vi "SRXConfigVoltageCompensation.vi"(3 "error in":errorcluster, 4 "RobotMotors":T16={"DriveRightPrimary"={"DeviceStatus"={"status"=FALSE, "code"=0, "source"=""}, "Type"=enum."PWM", "PWM"={"PWM Channel"=enum."PWM 1", "DeadBand"={"Name"="", "maxPositivePwm"=0, "minPositivePwm"=0, "centerPwm"=0, "maxNegativePwm"=0, "minNegativePwm"=0, "angularRange"=0}}, "CAN"={"Device Number"=0, "SetOutput VI Ref"=variant(enum8{"Percent VBus", "Current", "Speed", "Position", "Voltage"} enum."Percent VBus"), "GetOutput VI Ref"=variant(refnum<k1> refnum), "Enable VI Ref"=variant(dbl 12.0), "Disable VI Ref"=variant(enum8{"Percent VBus", "Speed", "Position", "Slave", "Unchanged / Invalid", "Voltage Compensation", "Current", "Motion Profile"} enum."Percent VBus"), "Data"=variant}, "Invert"=FALSE, "DIO PWM"={"PWM \"Enable\" Channel"=enum."Invalid", "DIOChannel"=enum."Invalid", "PWM Rate"=0.0}}, "DriveRightSecondary"={"DeviceStatus"={"status"=FALSE, "code"=0, "source"=""}, "Type"=enum."PWM", "PWM"={"PWM Channel"=enum."PWM 1", "DeadBand"={"Name"="", "maxPositivePwm"=0, "minPositivePwm"=0, "centerPwm"=0, "maxNegativePwm"=0, "minNegativePwm"=0, "angularRange"=0}}, "CAN"={"Device Number"=0, "SetOutput VI Ref"=variant(enum8{"Percent VBus", "Current", "Speed", "Position", "Voltage"} enum."Percent VBus"), "GetOutput VI Ref"=variant(refnum<k1> refnum), "Enable VI Ref"=variant(dbl 12.0), "Disable VI Ref"=variant(enum8{"Percent VBus", "Speed", "Position", "Slave", "Unchanged / Invalid", "Voltage Compensation", "Current", "Motion Profile"} enum."Percent VBus"), "Data"=variant}, "Invert"=FALSE, "DIO PWM"={"PWM \"Enable\" Channel"=enum."Invalid", "DIOChannel"=enum."Invalid", "PWM Rate"=0.0}}, "DriveLeftPrimary"={"DeviceStatus"={"status"=FALSE, "code"=0, "source"=""}, "Type"=enum."PWM", "PWM"={"PWM Channel"=enum."PWM 1", "DeadBand"={"Name"="", "maxPositivePwm"=0, "minPositivePwm"=0, "centerPwm"=0, "maxNegativePwm"=0, "minNegativePwm"=0, "angularRange"=0}}, "CAN"={"Device Number"=0, "SetOutput VI Ref"=variant(enum8{"Percent VBus", "Current", "Speed", "Position", "Voltage"} enum."Percent VBus"), "GetOutput VI Ref"=variant(refnum<k1> refnum), "Enable VI Ref"=variant(dbl 12.0), "Disable VI Ref"=variant(enum8{"Percent VBus", "Speed", "Position", "Slave", "Unchanged / Invalid", "Voltage Compensation", "Current", "Motion Profile"} enum."Percent VBus"), "Data"=variant}, "Invert"=FALSE, "DIO PWM"={"PWM \"Enable\" Channel"=enum."Invalid", "DIOChannel"=enum."Invalid", "PWM Rate"=0.0}}, "DriveLeftSecondary"={"DeviceStatus"={"status"=FALSE, "code"=0, "source"=""}, "Type"=enum."PWM", "PWM"={"PWM Channel"=enum."PWM 1", "DeadBand"={"Name"="", "maxPositivePwm"=0, "minPositivePwm"=0, "centerPwm"=0, "maxNegativePwm"=0, "minNegativePwm"=0, "angularRange"=0}}, "CAN"={"Device Number"=0, "SetOutput VI Ref"=variant(enum8{"Percent VBus", "Current", "Speed", "Position", "Voltage"} enum."Percent VBus"), "GetOutput VI Ref"=variant(refnum<k1> refnum), "Enable VI Ref"=variant(dbl 12.0), "Disable VI Ref"=variant(enum8{"Percent VBus", "Speed", "Position", "Slave", "Unchanged / Invalid", "Voltage Compensation", "Current", "Motion Profile"} enum."Percent VBus"), "Data"=variant}, "Invert"=FALSE, "DIO PWM"={"PWM \"Enable\" Channel"=enum."Invalid", "DIOChannel"=enum."Invalid", "PWM Rate"=0.0}}, " RearClimb"={"DeviceStatus"={"status"=FALSE, "code"=0, "source"=""}, "Type"=enum."PWM", "PWM"={"PWM Channel"=enum."PWM 1", "DeadBand"={"Name"="", "maxPositivePwm"=0, "minPositivePwm"=0, "centerPwm"=0, "maxNegativePwm"=0, "minNegativePwm"=0, "angularRange"=0}}, "CAN"={"Device Number"=0, "SetOutput VI Ref"=variant(enum8{"Percent VBus", "Current", "Speed", "Position", "Voltage"} enum."Percent VBus"), "GetOutput VI Ref"=variant(refnum<k1> refnum), "Enable VI Ref"=variant(dbl 12.0), "Disable VI Ref"=variant(enum8{"Percent VBus", "Speed", "Position", "Slave", "Unchanged / Invalid", "Voltage Compensation", "Current", "Motion Profile"} enum."Percent VBus"), "Data"=variant}, "Invert"=FALSE, "DIO PWM"={"PWM \"Enable\" Channel"=enum."Invalid", "DIOChannel"=enum."Invalid", "PWM Rate"=0.0}}, "FrontClimb"={"DeviceStatus"={"status"=FALSE, "code"=0, "source"=""}, "Type"=enum."PWM", "PWM"={"PWM Channel"=enum."PWM 1", "DeadBand"={"Name"="", "maxPositivePwm"=0, "minPositivePwm"=0, "centerPwm"=0, "maxNegativePwm"=0, "minNegativePwm"=0, "angularRange"=0}}, "CAN"={"Device Number"=0, "SetOutput VI Ref"=variant(enum8{"Percent VBus", "Current", "Speed", "Position", "Voltage"} enum."Percent VBus"), "GetOutput VI Ref"=variant(refnum<k1> refnum), "Enable VI Ref"=variant(dbl 12.0), "Disable VI Ref"=variant(enum8{"Percent VBus", "Speed", "Position", "Slave", "Unchanged / Invalid", "Voltage Compensation", "Current", "Motion Profile"} enum."Percent VBus"), "Data"=variant}, "Invert"=FALSE, "DIO PWM"={"PWM \"Enable\" Channel"=enum."Invalid", "DIOChannel"=enum."Invalid", "PWM Rate"=0.0}}, "ClimbDrive"={"DeviceStatus"={"status"=FALSE, "code"=0, "source"=""}, "Type"=enum."PWM", "PWM"={"PWM Channel"=enum."PWM 1", "DeadBand"={"Name"="", "maxPositivePwm"=0, "minPositivePwm"=0, "centerPwm"=0, "maxNegativePwm"=0, "minNegativePwm"=0, "angularRange"=0}}, "CAN"={"Device Number"=0, "SetOutput VI Ref"=variant(enum8{"Percent VBus", "Current", "Speed", "Position", "Voltage"} enum."Percent VBus"), "GetOutput VI Ref"=variant(refnum<k1> refnum), "Enable VI Ref"=variant(dbl 12.0), "Disable VI Ref"=variant(enum8{"Percent VBus", "Speed", "Position", "Slave", "Unchanged / Invalid", "Voltage Compensation", "Current", "Motion Profile"} enum."Percent VBus"), "Data"=variant}, "Invert"=FALSE, "DIO PWM"={"PWM \"Enable\" Channel"=enum."Invalid", "DIOChannel"=enum."Invalid", "PWM Rate"=0.0}}, "Shoulder2"={"DeviceStatus"={"status"=FALSE, "code"=0, "source"=""}, "Type"=enum."PWM", "PWM"={"PWM Channel"=enum."PWM 1", "DeadBand"={"Name"="", "maxPositivePwm"=0, "minPositivePwm"=0, "centerPwm"=0, "maxNegativePwm"=0, "minNegativePwm"=0, "angularRange"=0}}, "CAN"={"Device Number"=0, "SetOutput VI Ref"=variant(enum8{"Percent VBus", "Current", "Speed", "Position", "Voltage"} enum."Percent VBus"), "GetOutput VI Ref"=variant(refnum<k1> refnum), "Enable VI Ref"=variant(dbl 12.0), "Disable VI Ref"=variant(enum8{"Percent VBus", "Speed", "Position", "Slave", "Unchanged / Invalid", "Voltage Compensation", "Current", "Motion Profile"} enum."Percent VBus"), "Data"=variant}, "Invert"=FALSE, "DIO PWM"={"PWM \"Enable\" Channel"=enum."Invalid", "DIOChannel"=enum."Invalid", "PWM Rate"=0.0}}, "Shoulder1 "={"DeviceStatus"={"status"=FALSE, "code"=0, "source"=""}, "Type"=enum."PWM", "PWM"={"PWM Channel"=enum."PWM 1", "DeadBand"={"Name"="", "maxPositivePwm"=0, "minPositivePwm"=0, "centerPwm"=0, "maxNegativePwm"=0, "minNegativePwm"=0, "angularRange"=0}}, "CAN"={"Device Number"=0, "SetOutput VI Ref"=variant(enum8{"Percent VBus", "Current", "Speed", "Position", "Voltage"} enum."Percent VBus"), "GetOutput VI Ref"=variant(refnum<k1> refnum), "Enable VI Ref"=variant(dbl 12.0), "Disable VI Ref"=variant(enum8{"Percent VBus", "Speed", "Position", "Slave", "Unchanged / Invalid", "Voltage Compensation", "Current", "Motion Profile"} enum."Percent VBus"), "Data"=variant}, "Invert"=FALSE, "DIO PWM"={"PWM \"Enable\" Channel"=enum."Invalid", "DIOChannel"=enum."Invalid", "PWM Rate"=0.0}}, "Wrist"={"DeviceStatus"={"status"=FALSE, "code"=0, "source"=""}, "Type"=enum."PWM", "PWM"={"PWM Channel"=enum."PWM 1", "DeadBand"={"Name"="", "maxPositivePwm"=0, "minPositivePwm"=0, "centerPwm"=0, "maxNegativePwm"=0, "minNegativePwm"=0, "angularRange"=0}}, "CAN"={"Device Number"=0, "SetOutput VI Ref"=variant(enum8{"Percent VBus", "Current", "Speed", "Position", "Voltage"} enum."Percent VBus"), "GetOutput VI Ref"=variant(refnum<k1> refnum), "Enable VI Ref"=variant(dbl 12.0), "Disable VI Ref"=variant(enum8{"Percent VBus", "Speed", "Position", "Slave", "Unchanged / Invalid", "Voltage Compensation", "Current", "Motion Profile"} enum."Percent VBus"), "Data"=variant}, "Invert"=FALSE, "DIO PWM"={"PWM \"Enable\" Channel"=enum."Invalid", "DIOChannel"=enum."Invalid", "PWM Rate"=0.0}}, "Extension"={"DeviceStatus"={"status"=FALSE, "code"=0, "source"=""}, "Type"=enum."PWM", "PWM"={"PWM Channel"=enum."PWM 1", "DeadBand"={"Name"="", "maxPositivePwm"=0, "minPositivePwm"=0, "centerPwm"=0, "maxNegativePwm"=0, "minNegativePwm"=0, "angularRange"=0}}, "CAN"={"Device Number"=0, "SetOutput VI Ref"=variant(enum8{"Percent VBus", "Current", "Speed", "Position", "Voltage"} enum."Percent VBus"), "GetOutput VI Ref"=variant(refnum<k1> refnum), "Enable VI Ref"=variant(dbl 12.0), "Disable VI Ref"=variant(enum8{"Percent VBus", "Speed", "Position", "Slave", "Unchanged / Invalid", "Voltage Compensation", "Current", "Motion Profile"} enum."Percent VBus"), "Data"=variant}, "Invert"=FALSE, "DIO PWM"={"PWM \"Enable\" Channel"=enum."Invalid", "DIOChannel"=enum."Invalid", "PWM Rate"=0.0}}, "CargoIntake"={"DeviceStatus"={"status"=FALSE, "code"=0, "source"=""}, "Type"=enum."PWM", "PWM"={"PWM Channel"=enum."PWM 1", "DeadBand"={"Name"="", "maxPositivePwm"=0, "minPositivePwm"=0, "centerPwm"=0, "maxNegativePwm"=0, "minNegativePwm"=0, "angularRange"=0}}, "CAN"={"Device Number"=0, "SetOutput VI Ref"=variant(enum8{"Percent VBus", "Current", "Speed", "Position", "Voltage"} enum."Percent VBus"), "GetOutput VI Ref"=variant(refnum<k1> refnum), "Enable VI Ref"=variant(dbl 12.0), "Disable VI Ref"=variant(enum8{"Percent VBus", "Speed", "Position", "Slave", "Unchanged / Invalid", "Voltage Compensation", "Current", "Motion Profile"} enum."Percent VBus"), "Data"=variant}, "Invert"=FALSE, "DIO PWM"={"PWM \"Enable\" Channel"=enum."Invalid", "DIOChannel"=enum."Invalid", "PWM Rate"=0.0}}, "Intake2"={"DeviceStatus"={"status"=FALSE, "code"=0, "source"=""}, "Type"=enum."PWM", "PWM"={"PWM Channel"=enum."PWM 1", "DeadBand"={"Name"="", "maxPositivePwm"=0, "minPositivePwm"=0, "centerPwm"=0, "maxNegativePwm"=0, "minNegativePwm"=0, "angularRange"=0}}, "CAN"={"Device Number"=0, "SetOutput VI Ref"=variant(enum8{"Percent VBus", "Current", "Speed", "Position", "Voltage"} enum."Percent VBus"), "GetOutput VI Ref"=variant(refnum<k1> refnum), "Enable VI Ref"=variant(dbl 12.0), "Disable VI Ref"=variant(enum8{"Percent VBus", "Speed", "Position", "Slave", "Unchanged / Invalid", "Voltage Compensation", "Current", "Motion Profile"} enum."Percent VBus"), "Data"=variant}, "Invert"=FALSE, "DIO PWM"={"PWM \"Enable\" Channel"=enum."Invalid", "DIOChannel"=enum."Invalid", "PWM Rate"=0.0}}}, 5 "RobotConfig":T1={"Motors"={"DriveRightPrimary"={"CAN Address"=0, "Invert"=FALSE, "InvertSensor"=FALSE, "Unit Conversion Factor"=0.0, "Brake Mode"=enum."Override to Brake", "Reverse Limt Switch Mode"=enum."Normally Closed", "Forward Limt Swith Mode"=enum."Normally Closed", "PWM Channel"=enum."Invalid", "Motor Controller Type"=enum."Talon SRX", "Peak Current (A)"=0, "Continuos Current (A)"=0, "Peak Duration (ms)"=0, "Current Limit Enable"=FALSE}, "DriveRightSecondary"={"CAN Address"=0, "Invert"=FALSE, "InvertSensor"=FALSE, "Unit Conversion Factor"=0.0, "Brake Mode"=enum."Override to Brake", "Reverse Limt Switch Mode"=enum."Normally Closed", "Forward Limt Swith Mode"=enum."Normally Closed", "PWM Channel"=enum."Invalid", "Motor Controller Type"=enum."Talon SRX", "Peak Current (A)"=0, "Continuos Current (A)"=0, "Peak Duration (ms)"=0, "Current Limit Enable"=FALSE}, "DriveLeftPrimary"={"CAN Address"=0, "Invert"=FALSE, "InvertSensor"=FALSE, "Unit Conversion Factor"=0.0, "Brake Mode"=enum."Override to Brake", "Reverse Limt Switch Mode"=enum."Normally Closed", "Forward Limt Swith Mode"=enum."Normally Closed", "PWM Channel"=enum."Invalid", "Motor Controller Type"=enum."Talon SRX", "Peak Current (A)"=0, "Continuos Current (A)"=0, "Peak Duration (ms)"=0, "Current Limit Enable"=FALSE}, "DriveLeftSecondary"={"CAN Address"=0, "Invert"=FALSE, "InvertSensor"=FALSE, "Unit Conversion Factor"=0.0, "Brake Mode"=enum."Override to Brake", "Reverse Limt Switch Mode"=enum."Normally Closed", "Forward Limt Swith Mode"=enum."Normally Closed", "PWM Channel"=enum."Invalid", "Motor Controller Type"=enum."Talon SRX", "Peak Current (A)"=0, "Continuos Current (A)"=0, "Peak Duration (ms)"=0, "Current Limit Enable"=FALSE}, "RearClimb"={"CAN Address"=0, "Invert"=FALSE, "InvertSensor"=FALSE, "Unit Conversion Factor"=0.0, "Brake Mode"=enum."Override to Brake", "Reverse Limt Switch Mode"=enum."Normally Closed", "Forward Limt Swith Mode"=enum."Normally Closed", "PWM Channel"=enum."Invalid", "Motor Controller Type"=enum."Talon SRX", "Peak Current (A)"=0, "Continuos Current (A)"=0, "Peak Duration (ms)"=0, "Current Limit Enable"=FALSE}, "Front Climb"={"CAN Address"=0, "Invert"=FALSE, "InvertSensor"=FALSE, "Unit Conversion Factor"=0.0, "Brake Mode"=enum."Override to Brake", "Reverse Limt Switch Mode"=enum."Normally Closed", "Forward Limt Swith Mode"=enum."Normally Closed", "PWM Channel"=enum."Invalid", "Motor Controller Type"=enum."Talon SRX", "Peak Current (A)"=0, "Continuos Current (A)"=0, "Peak Duration (ms)"=0, "Current Limit Enable"=FALSE}, "Climb Drive"={"CAN Address"=0, "Invert"=FALSE, "InvertSensor"=FALSE, "Unit Conversion Factor"=0.0, "Brake Mode"=enum."Override to Brake", "Reverse Limt Switch Mode"=enum."Normally Closed", "Forward Limt Swith Mode"=enum."Normally Closed", "PWM Channel"=enum."Invalid", "Motor Controller Type"=enum."Talon SRX", "Peak Current (A)"=0, "Continuos Current (A)"=0, "Peak Duration (ms)"=0, "Current Limit Enable"=FALSE}, "Shoulder1"={"CAN Address"=0, "Invert"=FALSE, "InvertSensor"=FALSE, "Unit Conversion Factor"=0.0, "Brake Mode"=enum."Override to Brake", "Reverse Limt Switch Mode"=enum."Normally Closed", "Forward Limt Swith Mode"=enum."Normally Closed", "PWM Channel"=enum."Invalid", "Motor Controller Type"=enum."Talon SRX", "Peak Current (A)"=0, "Continuos Current (A)"=0, "Peak Duration (ms)"=0, "Current Limit Enable"=FALSE}, "Shoulder2"={"CAN Address"=9, "Invert"=FALSE, "InvertSensor"=FALSE, "Unit Conversion Factor"=0.0, "Brake Mode"=enum."Override to Brake", "Reverse Limt Switch Mode"=enum."Normally Closed", "Forward Limt Swith Mode"=enum."Normally Closed", "PWM Channel"=enum."Invalid", "Motor Controller Type"=enum."Talon SRX", "Peak Current (A)"=0, "Continuos Current (A)"=0, "Peak Duration (ms)"=0, "Current Limit Enable"=FALSE}, "Wrist"={"CAN Address"=10, "Invert"=FALSE, "InvertSensor"=FALSE, "Unit Conversion Factor"=0.0, "Brake Mode"=enum."Override to Brake", "Reverse Limt Switch Mode"=enum."Disabled", "Forward Limt Swith Mode"=enum."Disabled", "PWM Channel"=enum."Invalid", "Motor Controller Type"=enum."Talon SRX", "Peak Current (A)"=0, "Continuos Current (A)"=0, "Peak Duration (ms)"=0, "Current Limit Enable"=FALSE}, "Extension"={"CAN Address"=11, "Invert"=FALSE, "InvertSensor"=FALSE, "Unit Conversion Factor"=0.0, "Brake Mode"=enum."Override to Brake", "Reverse Limt Switch Mode"=enum."Disabled", "Forward Limt Swith Mode"=enum."Disabled", "PWM Channel"=enum."Invalid", "Motor Controller Type"=enum."Talon SRX", "Peak Current (A)"=0, "Continuos Current (A)"=0, "Peak Duration (ms)"=0, "Current Limit Enable"=FALSE}, "CargoIntake"={"CAN Address"=11, "Invert"=FALSE, "InvertSensor"=FALSE, "Unit Conversion Factor"=0.0, "Brake Mode"=enum."Override to Brake", "Reverse Limt Switch Mode"=enum."Disabled", "Forward Limt Swith Mode"=enum."Disabled", "PWM Channel"=enum."Invalid", "Motor Controller Type"=enum."Talon SRX", "Peak Current (A)"=0, "Continuos Current (A)"=0, "Peak Duration (ms)"=0, "Current Limit Enable"=FALSE}, "Intake2"={"CAN Address"=11, "Invert"=FALSE, "InvertSensor"=FALSE, "Unit Conversion Factor"=0.0, "Brake Mode"=enum."Override to Brake", "Reverse Limt Switch Mode"=enum."Disabled", "Forward Limt Swith Mode"=enum."Disabled", "PWM Channel"=enum."Invalid", "Motor Controller Type"=enum."Talon SRX", "Peak Current (A)"=0, "Continuos Current (A)"=0, "Peak Duration (ms)"=0, "Current Limit Enable"=FALSE}}, "Sensors"={"IMU"={"Yaw Axis"=enum."Z", "SPI Bus"=enum."SPI MXP", "AHRS Algorithm"=enum."Complementary", "Calibration Time (s)"=3.0, "Calibrate On Open"=TRUE}}, "PID"={"FrontClimb"={"P"=0.0, "I"=0.0, "D"=0.0, "F"=0.0, "IZone"=0.0}, "RearClimb"={"P"=0.0, "I"=0.0, "D"=0.0, "F"=0.0, "IZone"=0.0}, "ArmShoulder"={"P"=0.0, "I"=0.0, "D"=0.0, "F"=0.0, "IZone"=0.0}, "ArmExtend"={"P"=0.0, "I"=0.0, "D"=0.0, "F"=0.0, "IZone"=0.0}, "ArmWrist"={"P"=0.0, "I"=0.0, "D"=0.0, "F"=0.0, "IZone"=0.0}}, "Solenoids"={" Shifter"={"SolenoidChannel"=enum."Solenoid 0", "Invert"=FALSE}, "Hatch Grip"={"SolenoidChannel"=enum."Solenoid 0", "Invert"=FALSE}, "Hatch Extend"={"SolenoidChannel"=enum."Solenoid 0", "Invert"=FALSE}, "Manipulator Slide"={"SolenoidChannel"=enum."Solenoid 0", "Invert"=FALSE}, "Hatch Floor Intake"={"SolenoidChannel"=enum."Solenoid 0", "Invert"=FALSE}}, "Enable Compressor"=TRUE, "MotionMagic"={"FrontClimbExtend"={"CruiseVelocity"=0, "Acceleration"=0}, "RearClimbExtend"={"CruiseVelocity"=0, "Acceleration"=0}, "FrontClimbRetract"={"CruiseVelocity"=0, "Acceleration"=0}, "RearClimbRetract"={"CruiseVelocity"=0, "Acceleration"=0}}, "RobotDimensions"={"Length (in)"=0.0, "Shoulder Height (in)"=0.0, "Frame Height (in)"=0.0, "Arm Center to Front of Robot (in)"=0.0, "Arm Min Extension (in)"=0.0, "Arm Max Extension (in)"=0.0}, "Arm Home Position"={"Radius (in)"=0.0, "ShoulderAngle (rad)"=0.0, "WristAngle (rad)"=0.0}, "Climb Home Position"={"Back Climb"=0.0, "Front Climb"=0.0}, "Climb Positions"={"Retract"=0.0, "Level 2"=0.0, "Level 3"=0.0}}) -> (0 "error out":errorcluster, 1 "RobotMotorsOut":T16={"DriveRightPrimary"={"DeviceStatus"={"status"=FALSE, "code"=0, "source"=""}, "Type"=enum."PWM", "PWM"={"PWM Channel"=enum."PWM 1", "DeadBand"={"Name"="", "maxPositivePwm"=0, "minPositivePwm"=0, "centerPwm"=0, "maxNegativePwm"=0, "minNegativePwm"=0, "angularRange"=0}}, "CAN"={"Device Number"=0, "SetOutput VI Ref"=variant(enum8{"Percent VBus", "Current", "Speed", "Position", "Voltage"} enum."Percent VBus"), "GetOutput VI Ref"=variant(refnum<k1> refnum), "Enable VI Ref"=variant(dbl 12.0), "Disable VI Ref"=variant(enum8{"Percent VBus", "Speed", "Position", "Slave", "Unchanged / Invalid", "Voltage Compensation", "Current", "Motion Profile"} enum."Percent VBus"), "Data"=variant}, "Invert"=FALSE, "DIO PWM"={"PWM \"Enable\" Channel"=enum."Invalid", "DIOChannel"=enum."Invalid", "PWM Rate"=0.0}}, "DriveRightSecondary"={"DeviceStatus"={"status"=FALSE, "code"=0, "source"=""}, "Type"=enum."PWM", "PWM"={"PWM Channel"=enum."PWM 1", "DeadBand"={"Name"="", "maxPositivePwm"=0, "minPositivePwm"=0, "centerPwm"=0, "maxNegativePwm"=0, "minNegativePwm"=0, "angularRange"=0}}, "CAN"={"Device Number"=0, "SetOutput VI Ref"=variant(enum8{"Percent VBus", "Current", "Speed", "Position", "Voltage"} enum."Percent VBus"), "GetOutput VI Ref"=variant(refnum<k1> refnum), "Enable VI Ref"=variant(dbl 12.0), "Disable VI Ref"=variant(enum8{"Percent VBus", "Speed", "Position", "Slave", "Unchanged / Invalid", "Voltage Compensation", "Current", "Motion Profile"} enum."Percent VBus"), "Data"=variant}, "Invert"=FALSE, "DIO PWM"={"PWM \"Enable\" Channel"=enum."Invalid", "DIOChannel"=enum."Invalid", "PWM Rate"=0.0}}, "DriveLeftPrimary"={"DeviceStatus"={"status"=FALSE, "code"=0, "source"=""}, "Type"=enum."PWM", "PWM"={"PWM Channel"=enum."PWM 1", "DeadBand"={"Name"="", "maxPositivePwm"=0, "minPositivePwm"=0, "centerPwm"=0, "maxNegativePwm"=0, "minNegativePwm"=0, "angularRange"=0}}, "CAN"={"Device Number"=0, "SetOutput VI Ref"=variant(enum8{"Percent VBus", "Current", "Speed", "Position", "Voltage"} enum."Percent VBus"), "GetOutput VI Ref"=variant(refnum<k1> refnum), "Enable VI Ref"=variant(dbl 12.0), "Disable VI Ref"=variant(enum8{"Percent VBus", "Speed", "Position", "Slave", "Unchanged / Invalid", "Voltage Compensation", "Current", "Motion Profile"} enum."Percent VBus"), "Data"=variant}, "Invert"=FALSE, "DIO PWM"={"PWM \"Enable\" Channel"=enum."Invalid", "DIOChannel"=enum."Invalid", "PWM Rate"=0.0}}, "DriveLeftSecondary"={"DeviceStatus"={"status"=FALSE, "code"=0, "source"=""}, "Type"=enum."PWM", "PWM"={"PWM Channel"=enum."PWM 1", "DeadBand"={"Name"="", "maxPositivePwm"=0, "minPositivePwm"=0, "centerPwm"=0, "maxNegativePwm"=0, "minNegativePwm"=0, "angularRange"=0}}, "CAN"={"Device Number"=0, "SetOutput VI Ref"=variant(enum8{"Percent VBus", "Current", "Speed", "Position", "Voltage"} enum."Percent VBus"), "GetOutput VI Ref"=variant(refnum<k1> refnum), "Enable VI Ref"=variant(dbl 12.0), "Disable VI Ref"=variant(enum8{"Percent VBus", "Speed", "Position", "Slave", "Unchanged / Invalid", "Voltage Compensation", "Current", "Motion Profile"} enum."Percent VBus"), "Data"=variant}, "Invert"=FALSE, "DIO PWM"={"PWM \"Enable\" Channel"=enum."Invalid", "DIOChannel"=enum."Invalid", "PWM Rate"=0.0}}, " RearClimb"={"DeviceStatus"={"status"=FALSE, "code"=0, "source"=""}, "Type"=enum."PWM", "PWM"={"PWM Channel"=enum."PWM 1", "DeadBand"={"Name"="", "maxPositivePwm"=0, "minPositivePwm"=0, "centerPwm"=0, "maxNegativePwm"=0, "minNegativePwm"=0, "angularRange"=0}}, "CAN"={"Device Number"=0, "SetOutput VI Ref"=variant(enum8{"Percent VBus", "Current", "Speed", "Position", "Voltage"} enum."Percent VBus"), "GetOutput VI Ref"=variant(refnum<k1> refnum), "Enable VI Ref"=variant(dbl 12.0), "Disable VI Ref"=variant(enum8{"Percent VBus", "Speed", "Position", "Slave", "Unchanged / Invalid", "Voltage Compensation", "Current", "Motion Profile"} enum."Percent VBus"), "Data"=variant}, "Invert"=FALSE, "DIO PWM"={"PWM \"Enable\" Channel"=enum."Invalid", "DIOChannel"=enum."Invalid", "PWM Rate"=0.0}}, "FrontClimb"={"DeviceStatus"={"status"=FALSE, "code"=0, "source"=""}, "Type"=enum."PWM", "PWM"={"PWM Channel"=enum."PWM 1", "DeadBand"={"Name"="", "maxPositivePwm"=0, "minPositivePwm"=0, "centerPwm"=0, "maxNegativePwm"=0, "minNegativePwm"=0, "angularRange"=0}}, "CAN"={"Device Number"=0, "SetOutput VI Ref"=variant(enum8{"Percent VBus", "Current", "Speed", "Position", "Voltage"} enum."Percent VBus"), "GetOutput VI Ref"=variant(refnum<k1> refnum), "Enable VI Ref"=variant(dbl 12.0), "Disable VI Ref"=variant(enum8{"Percent VBus", "Speed", "Position", "Slave", "Unchanged / Invalid", "Voltage Compensation", "Current", "Motion Profile"} enum."Percent VBus"), "Data"=variant}, "Invert"=FALSE, "DIO PWM"={"PWM \"Enable\" Channel"=enum."Invalid", "DIOChannel"=enum."Invalid", "PWM Rate"=0.0}}, "ClimbDrive"={"DeviceStatus"={"status"=FALSE, "code"=0, "source"=""}, "Type"=enum."PWM", "PWM"={"PWM Channel"=enum."PWM 1", "DeadBand"={"Name"="", "maxPositivePwm"=0, "minPositivePwm"=0, "centerPwm"=0, "maxNegativePwm"=0, "minNegativePwm"=0, "angularRange"=0}}, "CAN"={"Device Number"=0, "SetOutput VI Ref"=variant(enum8{"Percent VBus", "Current", "Speed", "Position", "Voltage"} enum."Percent VBus"), "GetOutput VI Ref"=variant(refnum<k1> refnum), "Enable VI Ref"=variant(dbl 12.0), "Disable VI Ref"=variant(enum8{"Percent VBus", "Speed", "Position", "Slave", "Unchanged / Invalid", "Voltage Compensation", "Current", "Motion Profile"} enum."Percent VBus"), "Data"=variant}, "Invert"=FALSE, "DIO PWM"={"PWM \"Enable\" Channel"=enum."Invalid", "DIOChannel"=enum."Invalid", "PWM Rate"=0.0}}, "Shoulder2"={"DeviceStatus"={"status"=FALSE, "code"=0, "source"=""}, "Type"=enum."PWM", "PWM"={"PWM Channel"=enum."PWM 1", "DeadBand"={"Name"="", "maxPositivePwm"=0, "minPositivePwm"=0, "centerPwm"=0, "maxNegativePwm"=0, "minNegativePwm"=0, "angularRange"=0}}, "CAN"={"Device Number"=0, "SetOutput VI Ref"=variant(enum8{"Percent VBus", "Current", "Speed", "Position", "Voltage"} enum."Percent VBus"), "GetOutput VI Ref"=variant(refnum<k1> refnum), "Enable VI Ref"=variant(dbl 12.0), "Disable VI Ref"=variant(enum8{"Percent VBus", "Speed", "Position", "Slave", "Unchanged / Invalid", "Voltage Compensation", "Current", "Motion Profile"} enum."Percent VBus"), "Data"=variant}, "Invert"=FALSE, "DIO PWM"={"PWM \"Enable\" Channel"=enum."Invalid", "DIOChannel"=enum."Invalid", "PWM Rate"=0.0}}, "Shoulder1 "={"DeviceStatus"={"status"=FALSE, "code"=0, "source"=""}, "Type"=enum."PWM", "PWM"={"PWM Channel"=enum."PWM 1", "DeadBand"={"Name"="", "maxPositivePwm"=0, "minPositivePwm"=0, "centerPwm"=0, "maxNegativePwm"=0, "minNegativePwm"=0, "angularRange"=0}}, "CAN"={"Device Number"=0, "SetOutput VI Ref"=variant(enum8{"Percent VBus", "Current", "Speed", "Position", "Voltage"} enum."Percent VBus"), "GetOutput VI Ref"=variant(refnum<k1> refnum), "Enable VI Ref"=variant(dbl 12.0), "Disable VI Ref"=variant(enum8{"Percent VBus", "Speed", "Position", "Slave", "Unchanged / Invalid", "Voltage Compensation", "Current", "Motion Profile"} enum."Percent VBus"), "Data"=variant}, "Invert"=FALSE, "DIO PWM"={"PWM \"Enable\" Channel"=enum."Invalid", "DIOChannel"=enum."Invalid", "PWM Rate"=0.0}}, "Wrist"={"DeviceStatus"={"status"=FALSE, "code"=0, "source"=""}, "Type"=enum."PWM", "PWM"={"PWM Channel"=enum."PWM 1", "DeadBand"={"Name"="", "maxPositivePwm"=0, "minPositivePwm"=0, "centerPwm"=0, "maxNegativePwm"=0, "minNegativePwm"=0, "angularRange"=0}}, "CAN"={"Device Number"=0, "SetOutput VI Ref"=variant(enum8{"Percent VBus", "Current", "Speed", "Position", "Voltage"} enum."Percent VBus"), "GetOutput VI Ref"=variant(refnum<k1> refnum), "Enable VI Ref"=variant(dbl 12.0), "Disable VI Ref"=variant(enum8{"Percent VBus", "Speed", "Position", "Slave", "Unchanged / Invalid", "Voltage Compensation", "Current", "Motion Profile"} enum."Percent VBus"), "Data"=variant}, "Invert"=FALSE, "DIO PWM"={"PWM \"Enable\" Channel"=enum."Invalid", "DIOChannel"=enum."Invalid", "PWM Rate"=0.0}}, "Extension"={"DeviceStatus"={"status"=FALSE, "code"=0, "source"=""}, "Type"=enum."PWM", "PWM"={"PWM Channel"=enum."PWM 1", "DeadBand"={"Name"="", "maxPositivePwm"=0, "minPositivePwm"=0, "centerPwm"=0, "maxNegativePwm"=0, "minNegativePwm"=0, "angularRange"=0}}, "CAN"={"Device Number"=0, "SetOutput VI Ref"=variant(enum8{"Percent VBus", "Current", "Speed", "Position", "Voltage"} enum."Percent VBus"), "GetOutput VI Ref"=variant(refnum<k1> refnum), "Enable VI Ref"=variant(dbl 12.0), "Disable VI Ref"=variant(enum8{"Percent VBus", "Speed", "Position", "Slave", "Unchanged / Invalid", "Voltage Compensation", "Current", "Motion Profile"} enum."Percent VBus"), "Data"=variant}, "Invert"=FALSE, "DIO PWM"={"PWM \"Enable\" Channel"=enum."Invalid", "DIOChannel"=enum."Invalid", "PWM Rate"=0.0}}, "CargoIntake"={"DeviceStatus"={"status"=FALSE, "code"=0, "source"=""}, "Type"=enum."PWM", "PWM"={"PWM Channel"=enum."PWM 1", "DeadBand"={"Name"="", "maxPositivePwm"=0, "minPositivePwm"=0, "centerPwm"=0, "maxNegativePwm"=0, "minNegativePwm"=0, "angularRange"=0}}, "CAN"={"Device Number"=0, "SetOutput VI Ref"=variant(enum8{"Percent VBus", "Current", "Speed", "Position", "Voltage"} enum."Percent VBus"), "GetOutput VI Ref"=variant(refnum<k1> refnum), "Enable VI Ref"=variant(dbl 12.0), "Disable VI Ref"=variant(enum8{"Percent VBus", "Speed", "Position", "Slave", "Unchanged / Invalid", "Voltage Compensation", "Current", "Motion Profile"} enum."Percent VBus"), "Data"=variant}, "Invert"=FALSE, "DIO PWM"={"PWM \"Enable\" Channel"=enum."Invalid", "DIOChannel"=enum."Invalid", "PWM Rate"=0.0}}, "Intake2"={"DeviceStatus"={"status"=FALSE, "code"=0, "source"=""}, "Type"=enum."PWM", "PWM"={"PWM Channel"=enum."PWM 1", "DeadBand"={"Name"="", "maxPositivePwm"=0, "minPositivePwm"=0, "centerPwm"=0, "maxNegativePwm"=0, "minNegativePwm"=0, "angularRange"=0}}, "CAN"={"Device Number"=0, "SetOutput VI Ref"=variant(enum8{"Percent VBus", "Current", "Speed", "Position", "Voltage"} enum."Percent VBus"), "GetOutput VI Ref"=variant(refnum<k1> refnum), "Enable VI Ref"=variant(dbl 12.0), "Disable VI Ref"=variant(enum8{"Percent VBus", "Speed", "Position", "Slave", "Unchanged / Invalid", "Voltage Compensation", "Current", "Motion Profile"} enum."Percent VBus"), "Data"=variant}, "Invert"=FALSE, "DIO PWM"={"PWM \"Enable\" Channel"=enum."Invalid", "DIOChannel"=enum."Invalid", "PWM Rate"=0.0}}}, 2 "RobotConfigOut":T1={"Motors"={"DriveRightPrimary"={"CAN Address"=0, "Invert"=FALSE, "InvertSensor"=FALSE, "Unit Conversion Factor"=0.0, "Brake Mode"=enum."Override to Brake", "Reverse Limt Switch Mode"=enum."Normally Closed", "Forward Limt Swith Mode"=enum."Normally Closed", "PWM Channel"=enum."Invalid", "Motor Controller Type"=enum."Talon SRX", "Peak Current (A)"=0, "Continuos Current (A)"=0, "Peak Duration (ms)"=0, "Current Limit Enable"=FALSE}, "DriveRightSecondary"={"CAN Address"=0, "Invert"=FALSE, "InvertSensor"=FALSE, "Unit Conversion Factor"=0.0, "Brake Mode"=enum."Override to Brake", "Reverse Limt Switch Mode"=enum."Normally Closed", "Forward Limt Swith Mode"=enum."Normally Closed", "PWM Channel"=enum."Invalid", "Motor Controller Type"=enum."Talon SRX", "Peak Current (A)"=0, "Continuos Current (A)"=0, "Peak Duration (ms)"=0, "Current Limit Enable"=FALSE}, "DriveLeftPrimary"={"CAN Address"=0, "Invert"=FALSE, "InvertSensor"=FALSE, "Unit Conversion Factor"=0.0, "Brake Mode"=enum."Override to Brake", "Reverse Limt Switch Mode"=enum."Normally Closed", "Forward Limt Swith Mode"=enum."Normally Closed", "PWM Channel"=enum."Invalid", "Motor Controller Type"=enum."Talon SRX", "Peak Current (A)"=0, "Continuos Current (A)"=0, "Peak Duration (ms)"=0, "Current Limit Enable"=FALSE}, "DriveLeftSecondary"={"CAN Address"=0, "Invert"=FALSE, "InvertSensor"=FALSE, "Unit Conversion Factor"=0.0, "Brake Mode"=enum."Override to Brake", "Reverse Limt Switch Mode"=enum."Normally Closed", "Forward Limt Swith Mode"=enum."Normally Closed", "PWM Channel"=enum."Invalid", "Motor Controller Type"=enum."Talon SRX", "Peak Current (A)"=0, "Continuos Current (A)"=0, "Peak Duration (ms)"=0, "Current Limit Enable"=FALSE}, "RearClimb"={"CAN Address"=0, "Invert"=FALSE, "InvertSensor"=FALSE, "Unit Conversion Factor"=0.0, "Brake Mode"=enum."Override to Brake", "Reverse Limt Switch Mode"=enum."Normally Closed", "Forward Limt Swith Mode"=enum."Normally Closed", "PWM Channel"=enum."Invalid", "Motor Controller Type"=enum."Talon SRX", "Peak Current (A)"=0, "Continuos Current (A)"=0, "Peak Duration (ms)"=0, "Current Limit Enable"=FALSE}, "Front Climb"={"CAN Address"=0, "Invert"=FALSE, "InvertSensor"=FALSE, "Unit Conversion Factor"=0.0, "Brake Mode"=enum."Override to Brake", "Reverse Limt Switch Mode"=enum."Normally Closed", "Forward Limt Swith Mode"=enum."Normally Closed", "PWM Channel"=enum."Invalid", "Motor Controller Type"=enum."Talon SRX", "Peak Current (A)"=0, "Continuos Current (A)"=0, "Peak Duration (ms)"=0, "Current Limit Enable"=FALSE}, "Climb Drive"={"CAN Address"=0, "Invert"=FALSE, "InvertSensor"=FALSE, "Unit Conversion Factor"=0.0, "Brake Mode"=enum."Override to Brake", "Reverse Limt Switch Mode"=enum."Normally Closed", "Forward Limt Swith Mode"=enum."Normally Closed", "PWM Channel"=enum."Invalid", "Motor Controller Type"=enum."Talon SRX", "Peak Current (A)"=0, "Continuos Current (A)"=0, "Peak Duration (ms)"=0, "Current Limit Enable"=FALSE}, "Shoulder1"={"CAN Address"=0, "Invert"=FALSE, "InvertSensor"=FALSE, "Unit Conversion Factor"=0.0, "Brake Mode"=enum."Override to Brake", "Reverse Limt Switch Mode"=enum."Normally Closed", "Forward Limt Swith Mode"=enum."Normally Closed", "PWM Channel"=enum."Invalid", "Motor Controller Type"=enum."Talon SRX", "Peak Current (A)"=0, "Continuos Current (A)"=0, "Peak Duration (ms)"=0, "Current Limit Enable"=FALSE}, "Shoulder2"={"CAN Address"=9, "Invert"=FALSE, "InvertSensor"=FALSE, "Unit Conversion Factor"=0.0, "Brake Mode"=enum."Override to Brake", "Reverse Limt Switch Mode"=enum."Normally Closed", "Forward Limt Swith Mode"=enum."Normally Closed", "PWM Channel"=enum."Invalid", "Motor Controller Type"=enum."Talon SRX", "Peak Current (A)"=0, "Continuos Current (A)"=0, "Peak Duration (ms)"=0, "Current Limit Enable"=FALSE}, "Wrist"={"CAN Address"=10, "Invert"=FALSE, "InvertSensor"=FALSE, "Unit Conversion Factor"=0.0, "Brake Mode"=enum."Override to Brake", "Reverse Limt Switch Mode"=enum."Disabled", "Forward Limt Swith Mode"=enum."Disabled", "PWM Channel"=enum."Invalid", "Motor Controller Type"=enum."Talon SRX", "Peak Current (A)"=0, "Continuos Current (A)"=0, "Peak Duration (ms)"=0, "Current Limit Enable"=FALSE}, "Extension"={"CAN Address"=11, "Invert"=FALSE, "InvertSensor"=FALSE, "Unit Conversion Factor"=0.0, "Brake Mode"=enum."Override to Brake", "Reverse Limt Switch Mode"=enum."Disabled", "Forward Limt Swith Mode"=enum."Disabled", "PWM Channel"=enum."Invalid", "Motor Controller Type"=enum."Talon SRX", "Peak Current (A)"=0, "Continuos Current (A)"=0, "Peak Duration (ms)"=0, "Current Limit Enable"=FALSE}, "CargoIntake"={"CAN Address"=11, "Invert"=FALSE, "InvertSensor"=FALSE, "Unit Conversion Factor"=0.0, "Brake Mode"=enum."Override to Brake", "Reverse Limt Switch Mode"=enum."Disabled", "Forward Limt Swith Mode"=enum."Disabled", "PWM Channel"=enum."Invalid", "Motor Controller Type"=enum."Talon SRX", "Peak Current (A)"=0, "Continuos Current (A)"=0, "Peak Duration (ms)"=0, "Current Limit Enable"=FALSE}, "Intake2"={"CAN Address"=11, "Invert"=FALSE, "InvertSensor"=FALSE, "Unit Conversion Factor"=0.0, "Brake Mode"=enum."Override to Brake", "Reverse Limt Switch Mode"=enum."Disabled", "Forward Limt Swith Mode"=enum."Disabled", "PWM Channel"=enum."Invalid", "Motor Controller Type"=enum."Talon SRX", "Peak Current (A)"=0, "Continuos Current (A)"=0, "Peak Duration (ms)"=0, "Current Limit Enable"=FALSE}}, "Sensors"={"IMU"={"Yaw Axis"=enum."Z", "SPI Bus"=enum."SPI MXP", "AHRS Algorithm"=enum."Complementary", "Calibration Time (s)"=3.0, "Calibrate On Open"=TRUE}}, "PID"={"FrontClimb"={"P"=0.0, "I"=0.0, "D"=0.0, "F"=0.0, "IZone"=0.0}, "RearClimb"={"P"=0.0, "I"=0.0, "D"=0.0, "F"=0.0, "IZone"=0.0}, "ArmShoulder"={"P"=0.0, "I"=0.0, "D"=0.0, "F"=0.0, "IZone"=0.0}, "ArmExtend"={"P"=0.0, "I"=0.0, "D"=0.0, "F"=0.0, "IZone"=0.0}, "ArmWrist"={"P"=0.0, "I"=0.0, "D"=0.0, "F"=0.0, "IZone"=0.0}}, "Solenoids"={" Shifter"={"SolenoidChannel"=enum."Solenoid 0", "Invert"=FALSE}, "Hatch Grip"={"SolenoidChannel"=enum."Solenoid 0", "Invert"=FALSE}, "Hatch Extend"={"SolenoidChannel"=enum."Solenoid 0", "Invert"=FALSE}, "Manipulator Slide"={"SolenoidChannel"=enum."Solenoid 0", "Invert"=FALSE}, "Hatch Floor Intake"={"SolenoidChannel"=enum."Solenoid 0", "Invert"=FALSE}}, "Enable Compressor"=TRUE, "MotionMagic"={"FrontClimbExtend"={"CruiseVelocity"=0, "Acceleration"=0}, "RearClimbExtend"={"CruiseVelocity"=0, "Acceleration"=0}, "FrontClimbRetract"={"CruiseVelocity"=0, "Acceleration"=0}, "RearClimbRetract"={"CruiseVelocity"=0, "Acceleration"=0}}, "RobotDimensions"={"Length (in)"=0.0, "Shoulder Height (in)"=0.0, "Frame Height (in)"=0.0, "Arm Center to Front of Robot (in)"=0.0, "Arm Min Extension (in)"=0.0, "Arm Max Extension (in)"=0.0}, "Arm Home Position"={"Radius (in)"=0.0, "ShoulderAngle (rad)"=0.0, "WristAngle (rad)"=0.0}, "Climb Home Position"={"Back Climb"=0.0, "Front Climb"=0.0}, "Climb Positions"={"Retract"=0.0, "Level 2"=0.0, "Level 3"=0.0}})   [LabVIEW 2018]
uses:
  TypeDefs/ConfigComponents/Config_Robot.ctl
  ArgosLib/Config/ConfigComponents/TypeDefs/Config_Motor.ctl
  <vilib>/Rock Robotics/WPI/ThirdParty/Phoenix-LabVIEW/Motor Controller/Controls/CTRE_Phoenix_MotorControl_NeutralMode.ctl
  <vilib>/Rock Robotics/WPI/ThirdParty/Phoenix-LabVIEW/Motor Controller/Controls/CTRE_Phoenix_MotorControl_LimitSwitchNormal.ctl
  <vilib>/Rock Robotics/SystemInterfaces/DIO/FPGA_DIOPWMChannel.ctl
  ArgosLib/Config/ConfigComponents/TypeDefs/Config_MotorCtrlType.ctl
  ArgosLib/Config/ConfigComponents/TypeDefs/Config_IMU.ctl
  <vilib>/Rock Robotics/SystemInterfaces/spilib/spi_bus.ctl
  ArgosLib/Config/ConfigComponents/TypeDefs/Config_PIDParams.ctl
  ArgosLib/Config/ConfigComponents/TypeDefs/Config_SingleSolenoid.ctl
  <vilib>/Rock Robotics/WPI/Solenoid/WPI_SolenoidChannel.ctl
  ArgosLib/Config/ConfigComponents/TypeDefs/Config_MotionMagicParams.ctl
  TypeDefs/ConfigComponents/Config_Dimensions.ctl
  Implements/Arm/TypeDefs/ArmCoordinate.ctl
  Implements/Climber/TypeDefs/ClimberPositionHeights.ctl
  TypeDefs/RobotComponents/RobotMotors.ctl
  <vilib>/Rock Robotics/WPI/MotorControl/WPI_MotorControlDeviceRef.ctl
  <vilib>/Rock Robotics/WPI/MotorControl/WPI_MotorControlType.ctl
  <vilib>/Rock Robotics/WPI/PWM/WPI_PWMDeadband.ctl
  <vilib>/Rock Robotics/SystemInterfaces/DIO/FPGA_DIOChannel.ctl
  ArgosLib/ArgosLib.lvlib
panel:
  in  "Saturation Voltage":dbl=11.5
  in  "Enable Voltage Compensation?":bool=TRUE
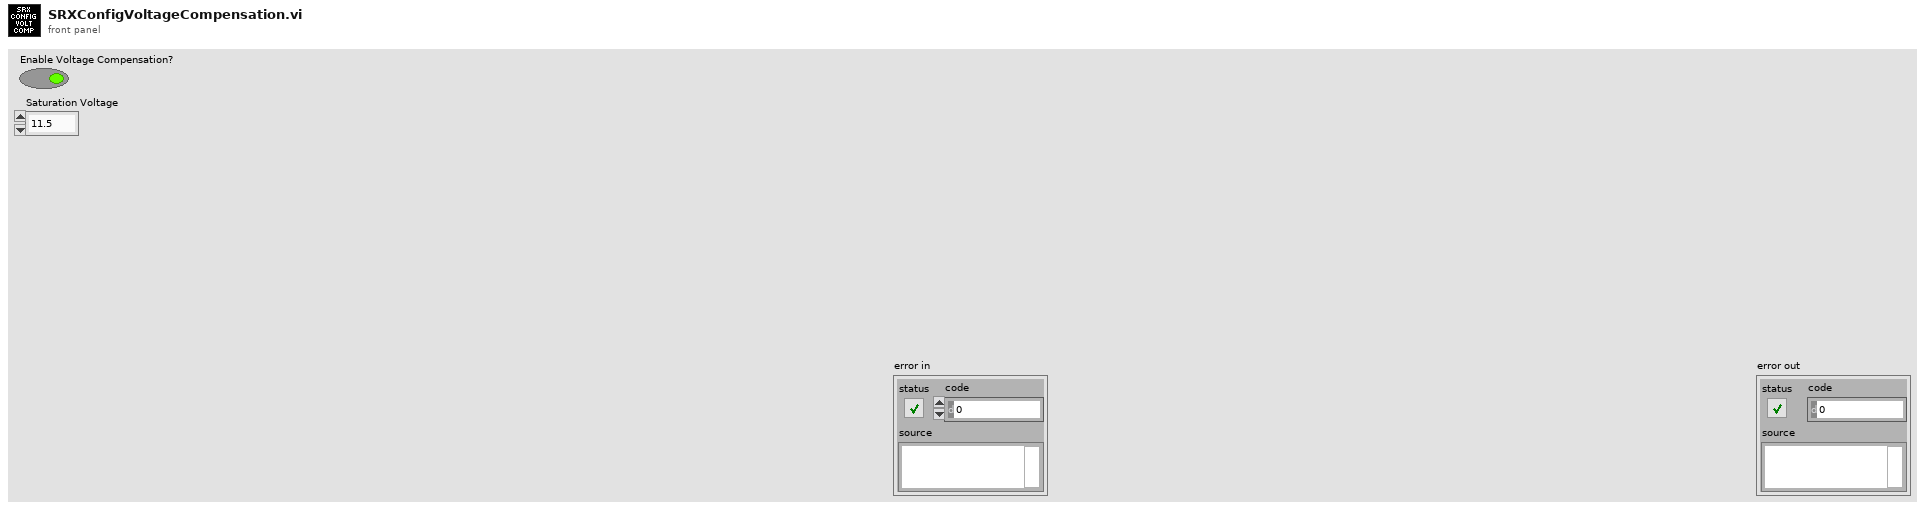
[diagram p1: front panel]
types:
  T1 = typedef "Config_Robot.ctl" = cluster{"Motors":cluster{"DriveRightPrimary":T2, "DriveRightSecondary":T2, "DriveLeftPrimary":T2, "DriveLeftSecondary":T2, "RearClimb":T2, "Front Climb":T2, "Climb Drive":T2, "Shoulder1":T2, "Shoulder2":T2, "Wrist":T2, "Extension":T2, "CargoIntake":T2, "Intake2":T2}, "Sensors":cluster{"IMU":T7}, "PID":cluster{"FrontClimb":T9, "RearClimb":T9, "ArmShoulder":T9, "ArmExtend":T9, "ArmWrist":T9}, "Solenoids":cluster{" Shifter":T10, "Hatch Grip":T10, "Hatch Extend":T10, "Manipulator Slide":T10, "Hatch Floor Intake":T10}, "Enable Compressor":bool, "MotionMagic":cluster{"FrontClimbExtend":T12, "RearClimbExtend":T12, "FrontClimbRetract":T12, "RearClimbRetract":T12}, "RobotDimensions":T13, "Arm Home Position":T14, "Climb Home Position":cluster{"Back Climb":dbl, "Front Climb":dbl}, "Climb Positions":T15}
  T2 = typedef "ArgosLib.lvlib/Config_Motor.ctl" = cluster{"CAN Address":u8, "Invert":bool, "InvertSensor":bool, "Unit Conversion Factor":dbl, "Brake Mode":T3, "Reverse Limt Switch Mode":T4, "Forward Limt Swith Mode":T4, "PWM Channel":T5, "Motor Controller Type":T6, "Peak Current (A)":i32, "Continuos Current (A)":i32, "Peak Duration (ms)":i32, "Current Limit Enable":bool}
  T3 = typedef "CTRE_Phoenix_MotorControl_NeutralMode.ctl" = enum8{"EEPROMSetting", "Override to Coast", "Override to Brake"}
  T4 = typedef "CTRE_Phoenix_MotorControl_LimitSwitchNormal.ctl" = enum16{"Normally Open", "Normally Closed", "Disabled"}
  T5 = typedef "FPGA_DIOPWMChannel.ctl" = enum8{"PWM 0", "PWM 1", "PWM 2", "PWM 3", "PWM 4", "PWM 5", "PWM 6", "PWM 7", "PWM 8", "PWM 9", "PWM MXP 0", "PWM MXP 1", "PWM MXP 2", "PWM MXP 3", "PWM MXP 4", "PWM MXP 5", "PWM MXP 6", "PWM MXP 7", "PWM MXP 8", "PWM MXP 9", "Invalid"}
  T6 = typedef "ArgosLib.lvlib/Config_MotorCtrlType.ctl" = enum16{"Disabled", "Talon SRX", "Talon SR"}
  T7 = typedef "ArgosLib.lvlib/Config_IMU.ctl" = cluster{"Yaw Axis":enum16{"X", "Y", "Z"}, "SPI Bus":T8, "AHRS Algorithm":enum16{"Complementary", "Madgwick"}, "Calibration Time (s)":dbl, "Calibrate On Open":bool}
  T8 = typedef "spi_bus.ctl" = enum16{"SPI On-Board, CS0", "SPI On-Board, CS1", "SPI On-Board, CS2", "SPI On-Board, CS3", "SPI MXP", "Invalid"}
  T9 = typedef "ArgosLib.lvlib/Config_PIDParams.ctl" = cluster{"P":dbl, "I":dbl, "D":dbl, "F":dbl, "IZone":dbl}
  T10 = typedef "ArgosLib.lvlib/Config_SingleSolenoid.ctl" = cluster{"SolenoidChannel":T11, "Invert":bool}
  T11 = typedef "WPI_SolenoidChannel.ctl" = enum8{"Solenoid 0", "Solenoid 1", "Solenoid 2", "Solenoid 3", "Solenoid 4", "Solenoid 5", "Solenoid 6", "Solenoid 7", "Invalid"}
  T12 = typedef "Config_MotionMagicParams.ctl" = cluster{"CruiseVelocity":i32, "Acceleration":i32}
  T13 = typedef "Config_Dimensions.ctl" = cluster{"Length (in)":dbl, "Shoulder Height (in)":dbl, "Frame Height (in)":dbl, "Arm Center to Front of Robot (in)":dbl, "Arm Min Extension (in)":dbl, "Arm Max Extension (in)":dbl}
  T14 = typedef "ArmCoordinate.ctl" = cluster{"Radius (in)":dbl, "ShoulderAngle (rad)":dbl, "WristAngle (rad)":dbl}
  T15 = typedef "ClimberPositionHeights.ctl" = cluster{"Retract":dbl, "Level 2":dbl, "Level 3":dbl}
  T16 = typedef "RobotMotors.ctl" = cluster{"DriveRightPrimary":T17, "DriveRightSecondary":T17, "DriveLeftPrimary":T17, "DriveLeftSecondary":T17, " RearClimb":T17, "FrontClimb":T17, "ClimbDrive":T17, "Shoulder2":T17, "Shoulder1 ":T17, "Wrist":T17, "Extension":T17, "CargoIntake":T17, "Intake2":T17}
  T17 = typedef "WPI_MotorControlDeviceRef.ctl" = cluster{"DeviceStatus":errorcluster, "Type":T18, "PWM":cluster{"PWM Channel":T5, "DeadBand":T19}, "CAN":cluster{"Device Number":u8, "SetOutput VI Ref":variant, "GetOutput VI Ref":variant, "Enable VI Ref":variant, "Disable VI Ref":variant, "Data":variant}, "Invert":bool, "DIO PWM":cluster{"PWM \"Enable\" Channel":T5, "DIOChannel":T20, "PWM Rate":dbl}}
  T18 = typedef "WPI_MotorControlType.ctl" = enum16{"PWM", "CAN", "DIO PWM"}
  T19 = typedef "WPI_PWMDeadband.ctl" = cluster{"Name":string, "maxPositivePwm":i32, "minPositivePwm":i32, "centerPwm":i32, "maxNegativePwm":i32, "minNegativePwm":i32, "angularRange":u16}
  T20 = typedef "FPGA_DIOChannel.ctl" = enum8{"DIO 0", "DIO 1", "DIO 2", "DIO 3", "DIO 4", "DIO 5", "DIO 6", "DIO 7", "DIO 8", "DIO 9", "DIO MXP 0", "DIO MXP 1", "DIO MXP 2", "DIO MXP 3", "DIO MXP 4", "DIO MXP 5", "DIO MXP 6", "DIO MXP 7", "DIO MXP 8", "DIO MXP 9", "DIO MXP 10", "DIO MXP 11", "DIO MXP 12", "DIO MXP 13", "DIO MXP 14", "DIO MXP 15", "SPI Port CS1", "SPI Port CS2", "SPI Port CS3", "SPI Port MISO", "SPI Port MOSI", "Invalid"}
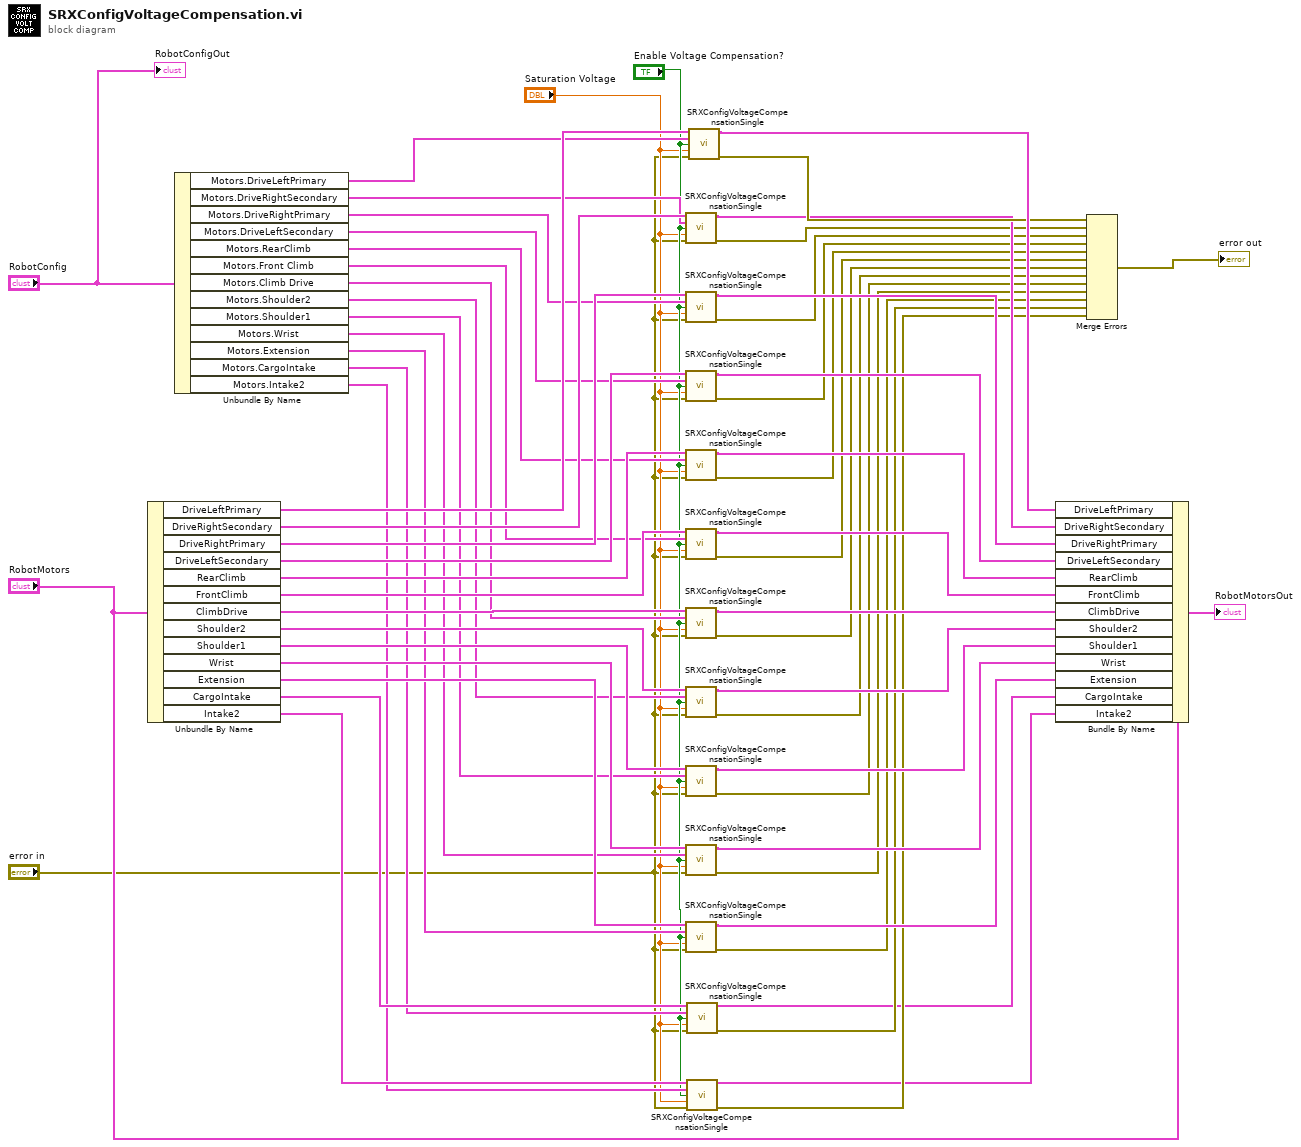
[diagram p0: block diagram]
diagram:
  n1 = Unbundle By Name("RobotMotors") -> ("DriveLeftPrimary"=w50:T17, "DriveRightSecondary"=w51:T17, "DriveRightPrimary"=w52:T17, "DriveLeftSecondary"=w53:T17, "RearClimb"=w54:T17, "FrontClimb"=w55:T17, "ClimbDrive"=w56:T17, "Shoulder2"=w57:T17, "Shoulder1"=w58:T17, "Wrist"=w59:T17, "Extension"=w46:T17, "CargoIntake"=w11:T17, "Intake2"=w10:T17)
  n2 = Unbundle By Name("RobotConfig") -> ("Motors.DriveLeftPrimary"=w44:T2, "Motors.DriveRightSecondary"=w43:T2, "Motors.DriveRightPrimary"=w42:T2, "Motors.DriveLeftSecondary"=w41:T2, "Motors.RearClimb"=w40:T2, "Motors.Front Climb"=w39:T2, "Motors.Climb Drive"=w38:T2, "Motors.Shoulder2"=w37:T2, "Motors.Shoulder1"=w36:T2, "Motors.Wrist"=w35:T2, "Motors.Extension"=w34:T2, "Motors.CargoIntake"=w9:T2, "Motors.Intake2"=w8:T2)
  n3 = call "SRXConfigVoltageCompensationSingle.vi"("PhoenixMotorControlDevRefIn"=w51, "MotorConfig"=w43, "Enable Voltage Compensation?"="Enable Voltage Compensation?", "Saturation Voltage"="Saturation Voltage", "error in (no error)"="error in") -> ("PhoenixMotorControlDevRefOut"=w31:T17, "error out"=w30:errorcluster)  [unwired: 9 in]
  n4 = call "SRXConfigVoltageCompensationSingle.vi"("PhoenixMotorControlDevRefIn"=w52, "MotorConfig"=w42, "Enable Voltage Compensation?"="Enable Voltage Compensation?", "Saturation Voltage"="Saturation Voltage", "error in (no error)"="error in") -> ("PhoenixMotorControlDevRefOut"=w29:T17, "error out"=w28:errorcluster)  [unwired: 9 in]
  n5 = call "SRXConfigVoltageCompensationSingle.vi"("PhoenixMotorControlDevRefIn"=w53, "MotorConfig"=w41, "Enable Voltage Compensation?"="Enable Voltage Compensation?", "Saturation Voltage"="Saturation Voltage", "error in (no error)"="error in") -> ("PhoenixMotorControlDevRefOut"=w27:T17, "error out"=w26:errorcluster)  [unwired: 9 in]
  n6 = call "SRXConfigVoltageCompensationSingle.vi"("PhoenixMotorControlDevRefIn"=w54, "MotorConfig"=w40, "Enable Voltage Compensation?"="Enable Voltage Compensation?", "Saturation Voltage"="Saturation Voltage", "error in (no error)"="error in") -> ("PhoenixMotorControlDevRefOut"=w25:T17, "error out"=w24:errorcluster)  [unwired: 9 in]
  n7 = call "SRXConfigVoltageCompensationSingle.vi"("PhoenixMotorControlDevRefIn"=w55, "MotorConfig"=w39, "Enable Voltage Compensation?"="Enable Voltage Compensation?", "Saturation Voltage"="Saturation Voltage", "error in (no error)"="error in") -> ("PhoenixMotorControlDevRefOut"=w23:T17, "error out"=w22:errorcluster)  [unwired: 9 in]
  n8 = call "SRXConfigVoltageCompensationSingle.vi"("PhoenixMotorControlDevRefIn"=w56, "MotorConfig"=w38, "Enable Voltage Compensation?"="Enable Voltage Compensation?", "Saturation Voltage"="Saturation Voltage", "error in (no error)"="error in") -> ("PhoenixMotorControlDevRefOut"=w21:T17, "error out"=w20:errorcluster)  [unwired: 9 in]
  n9 = call "SRXConfigVoltageCompensationSingle.vi"("PhoenixMotorControlDevRefIn"=w57, "MotorConfig"=w37, "Enable Voltage Compensation?"="Enable Voltage Compensation?", "Saturation Voltage"="Saturation Voltage", "error in (no error)"="error in") -> ("PhoenixMotorControlDevRefOut"=w19:T17, "error out"=w18:errorcluster)  [unwired: 9 in]
  n10 = call "SRXConfigVoltageCompensationSingle.vi"("PhoenixMotorControlDevRefIn"=w58, "MotorConfig"=w36, "Enable Voltage Compensation?"="Enable Voltage Compensation?", "Saturation Voltage"="Saturation Voltage", "error in (no error)"="error in") -> ("PhoenixMotorControlDevRefOut"=w17:T17, "error out"=w16:errorcluster)  [unwired: 9 in]
  n11 = call "SRXConfigVoltageCompensationSingle.vi"("PhoenixMotorControlDevRefIn"=w59, "MotorConfig"=w35, "Enable Voltage Compensation?"="Enable Voltage Compensation?", "Saturation Voltage"="Saturation Voltage", "error in (no error)"="error in") -> ("PhoenixMotorControlDevRefOut"=w15:T17, "error out"=w14:errorcluster)  [unwired: 9 in]
  n12 = call "SRXConfigVoltageCompensationSingle.vi"("PhoenixMotorControlDevRefIn"=w46, "MotorConfig"=w34, "Enable Voltage Compensation?"="Enable Voltage Compensation?", "Saturation Voltage"="Saturation Voltage", "error in (no error)"="error in") -> ("PhoenixMotorControlDevRefOut"=w13:T17, "error out"=w12:errorcluster)  [unwired: 9 in]
  n13 = call "SRXConfigVoltageCompensationSingle.vi"("PhoenixMotorControlDevRefIn"=w11, "MotorConfig"=w9, "Enable Voltage Compensation?"="Enable Voltage Compensation?", "Saturation Voltage"="Saturation Voltage", "error in (no error)"="error in") -> ("PhoenixMotorControlDevRefOut"=w2:T17, "error out"=w4:errorcluster)  [unwired: 9 in]
  n14 = call "SRXConfigVoltageCompensationSingle.vi"("PhoenixMotorControlDevRefIn"=w10, "MotorConfig"=w8, "Enable Voltage Compensation?"="Enable Voltage Compensation?", "Saturation Voltage"="Saturation Voltage", "error in (no error)"="error in") -> ("PhoenixMotorControlDevRefOut"=w1:T17, "error out"=w3:errorcluster)  [unwired: 9 in]
  n15 = call "SRXConfigVoltageCompensationSingle.vi"("PhoenixMotorControlDevRefIn"=w50, "MotorConfig"=w44, "Enable Voltage Compensation?"="Enable Voltage Compensation?", "Saturation Voltage"="Saturation Voltage", "error in (no error)"="error in") -> ("PhoenixMotorControlDevRefOut"=w33:T17, "error out"=w32:errorcluster)  [unwired: 9 in]
  n16 = Bundle By Name(cluster="RobotMotors", "DriveLeftPrimary"=w33, "DriveRightSecondary"=w31, "DriveRightPrimary"=w29, "DriveLeftSecondary"=w27, "RearClimb"=w25, "FrontClimb"=w23, "ClimbDrive"=w21, "Shoulder2"=w19, "Shoulder1"=w17, "Wrist"=w15, "Extension"=w13, "CargoIntake"=w2, "Intake2"=w1) -> (→"RobotMotorsOut":T16)
  n17 = Merge Errors(w32, w30, w28, w26, w24, w22, w20, w18, w16, w14, w12, w4, w3) -> (→"error out":errorcluster)
  "RobotConfigOut" <- "RobotConfig"
